vi "teacherTimer.vi"(6 "Timer action (Get Time)":T1, 8 "error in (no error)":errorcluster, 11 "Time to elapse":dbl) -> (0 "error out":errorcluster, 1 "Time elapsed":bool, 3 "Current time":dbl)   [LabVIEW 2022 SP3]
doc: "This VI elapses time"
uses:
  teacherTimer_action.ctl
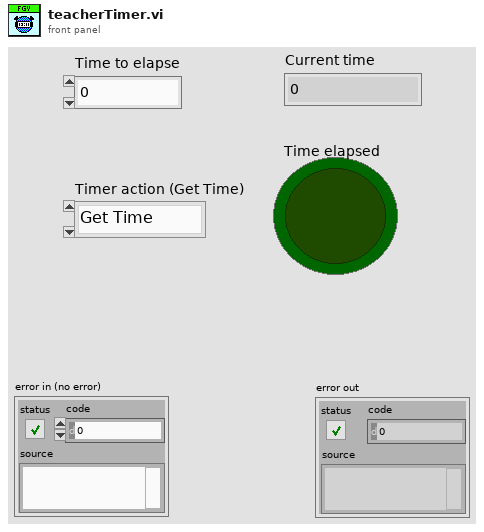
[diagram p1: front panel]
types:
  T1 = typedef "teacherTimer_action.ctl" = enum16{"Get Time", "Reset"}
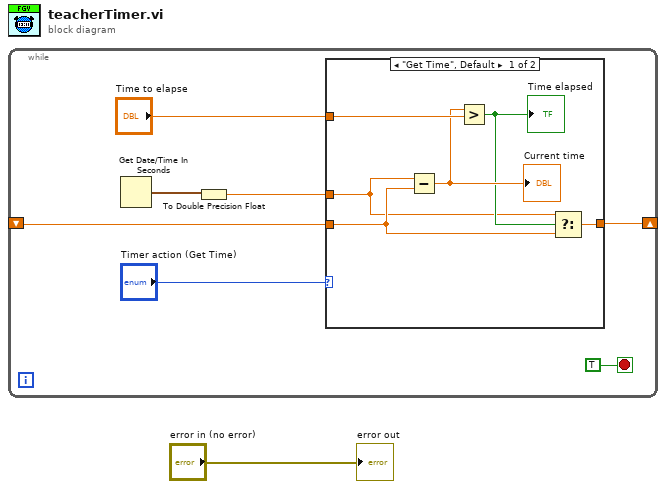
[diagram p0: block diagram]
diagram:
  n1 = while {
    shift-right: [w4] -> _
    shift-left: _ -> [w5]
    stop <- TRUE stop-if-true
    n2 = Get Date/Time In Seconds() -> (seconds since 1Jan1904=w7:timestamp)
    n3 = To Double Precision Float(number=w7) -> (double precision float=w6:dbl)
    n4 = case shown="\"Get Time\", Default" "Timer action (Get Time)" {
      tunnel: w6 -> [w9 w15]
      tunnel: w5 -> [w10 _]
      tunnel: [w12 w15] -> w4
      tunnel: "Time to elapse" -> [w14 _]
      frame "Get Time", Default {
        n5 = Subtract(x=w9, y=w10) -> (x-y=w13:dbl)
        "Current time" <- w13
        n6 = Greater?(x=w13, y=w14) -> (0:w11:bool)
        "Time elapsed" <- w11
        n7 = Select(t=w9, s=w11, f=w10) -> (s? t:f=w12:dbl)
      }
      frame "Reset" {
      }
    }
  }
  "error out" <- "error in (no error)"
